vi "FTW-Ether-Address-RandomEphemeral.vi"(5 "Endpoint":T1, 11 "error in":errorcluster) -> (6 "Endpoint with Replacements":T1, 15 "error out":errorcluster)   [LabVIEW 2012, in "FTW-Actor.lvlib" / "FTW-Ether.lvclass"]
uses:
  FTW-Ether.lvclass
  Utility/FTW-Actor-Address.ctl
  FTW-Actor.lvlib
panel:
  # "Inputs"
  # "Outputs"
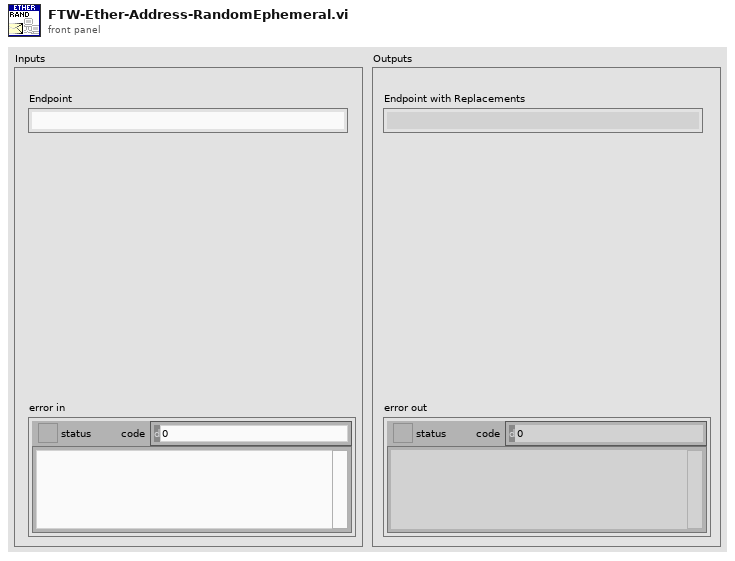
[diagram p1: front panel]
types:
  T1 = typedef "FTW-Actor.lvlib/FTW-Actor-Address.ctl" = string
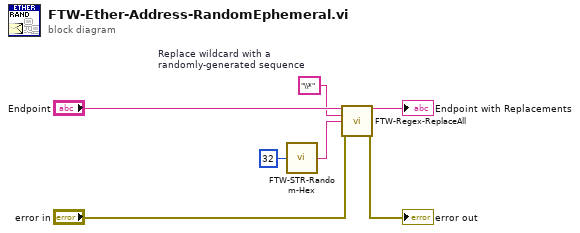
[diagram p0: block diagram]
diagram:
  w3 = "\\*"  # Replace wildcard with a randomly-generated sequence
  n1 = call "FTW-STR-Random-Hex.vi"("String Length"=32) -> ("Random Hex String"=w1:string)  [unwired: 3 in]
  n2 = call "FTW-Regex-ReplaceAll.vi"("String"="Endpoint", "Search for (Regular Expression)"=w3, "Replace with"=w1, "error in"="error in") -> ("String out"=→"Endpoint with Replacements":string, "error out"=→"error out":errorcluster)  [unwired: 9 in, 1 out]
